vi "ff init.vi"(4 "pix_fmt_in":i32, 5 "fps":i32=30, 6 "bit_rate":i32, 7 "height":i32, 9 "width":i32, 10 "codec_id":i32=28, 11 "filename":string) -> (3 "function return":i32)   [LabVIEW 2013, in "ffvi.lvlib"]
doc: "int ff_init(const char *filename, \n int codec_id, \n int width, \n int height, \n int bit_rate,\n int fps,\n int pix_fmt);"
uses:
  ffvi.lvlib
  ffvi.dll
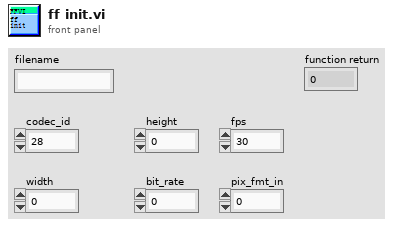
[diagram p1: front panel]
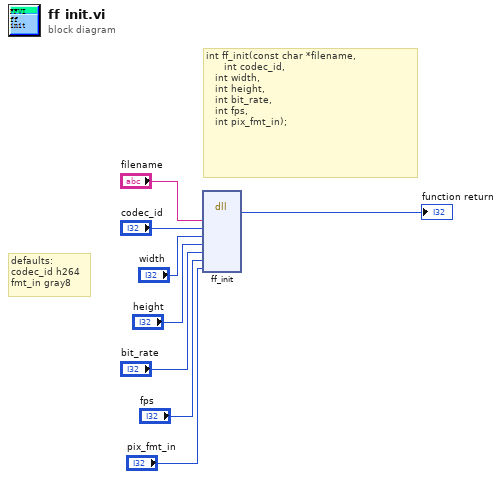
[diagram p0: block diagram]
diagram:
  # "defaults:\ncodec_id h264\nfmt_in gray8"
  # "int ff_init(const char *filename, \n\t\t    int codec_id, \n\t\t\tint width, \n\t\t\tint height, \n\t\t\tint bit_rate,\n\t\t\tint fps,\n\t\t\tint pix_fmt_in);"
  n1 = dll-call lib="D:/ffmpeg/ffvi/ffvi.*" fn="ff_init"("filename"="filename", "codec_id"="codec_id", "width"="width", "height"="height", "bit_rate"="bit_rate", "fps"="fps", "pix_fmt_in"="pix_fmt_in") -> ("return type"=→"function return":i32)  [unwired: 10 in, 2 out]
